vi "Temp_global_BM.vi"() -> ()   [LabVIEW 2021]
panel:
  out "Final Temp (oC)":dbl
  out "Max Temp (oC)":dbl
  out "Intial Temp (oC)":dbl
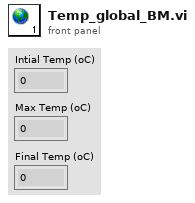
[diagram p1: front panel]
diagram:
